vi "StartController.vi"(8 "error in (no error)":errorcluster, 11 "Panel_UI in":refnum<class "Panel_UI.lvclass">) -> (0 "error out":errorcluster, 3 "Panel_UI out":refnum<class "Panel_UI.lvclass">)   [LabVIEW 2015, in "Panel_UI.lvclass"]
uses:
  Panel_UI.lvclass
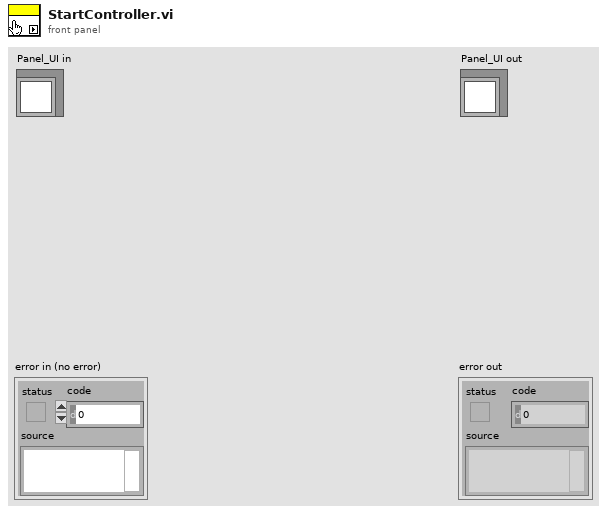
[diagram p1: front panel]
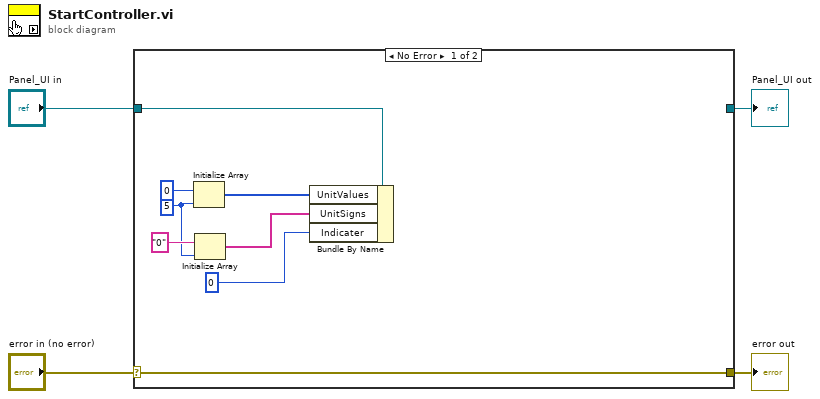
[diagram p0: block diagram]
diagram:
  n1 = case shown="No Error" "error in (no error)" {
    selector: "error in (no error)" -> [w13 w15]
    tunnel: [w13 w15] -> w3
    tunnel: [w5 w14] -> w1
    tunnel: "Panel_UI in" -> [w12 w14]
    frame No Error {
      w8 = 5 ("dimension size")
      n2 = Initialize Array(0, w8) -> (w10:i32[])
      n3 = Initialize Array("0", w8) -> (w7:string[])
      n4 = Bundle By Name(cluster=w12, "UnitValues"=w10, "UnitSigns"=w7, "Indicater"=0) -> ()  [unwired: 1 out]
    }
    frame Error {
    }
  }
  "error out" <- w3
  "Panel_UI out" <- w1
